vi "Date_request.vi"(8 "error in (no error)":errorcluster, 10 "SQL request":string, 11 "DB_SQLite in":refnum<class "DB_SQLite.lvclass">) -> (0 "error out":errorcluster, 2 "Date":timestamp, 3 "DB_SQLite out":refnum<class "DB_SQLite.lvclass">)   [LabVIEW 2015, in "DB_SQLite.lvclass"]
uses:
  DB_SQLite.lvclass
  <vilib>/drjdpowell/SQLite Library/SQL Connection/Connection.lvclass
  <vilib>/drjdpowell/SQLite Library/SQL Connection/Open (path).vi
  <vilib>/drjdpowell/SQLite Library/SQLite.lvlib
  DB.lvclass
  <vilib>/drjdpowell/SQLite Library/SQL Connection/Execute SQL (No results).vi
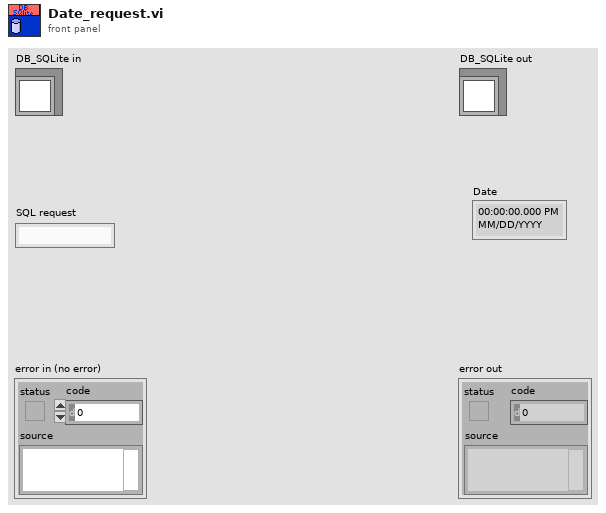
[diagram p1: front panel]
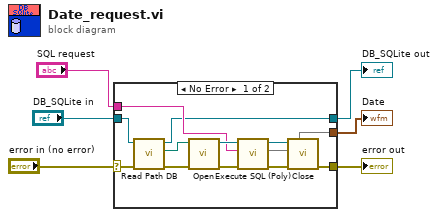
[diagram p0: block diagram]
diagram:
  n1 = case shown="No Error" "error in (no error)" {
    selector: "error in (no error)" -> [w10 w19]
    tunnel: [w7 w20] -> w5
    tunnel: "DB_SQLite in" -> [w11 w20]
    tunnel: "SQL request" -> [w14 _]
    tunnel: [w13 _] -> w2
    tunnel: [w12 w19] -> w1
    frame No Error {
      n2 = call "Read Path DB.vi"("error in (no error)"=w10, "DB in"=w11) -> ("error out"=w9:errorcluster, "Path DB"=w8:path, "DB out"=w7:refnum<class "DB_SQLite.lvclass">)  [unwired: 7 in]
      n3 = call-poly <vilib>:"Open.vi"("error in (no error)"=w9, "db file"=w8) -> ("error out"=w15:errorcluster, "SQLite Connection"=w16:refnum<class "Connection.lvclass">)  [unwired: 8 in]
      n4 = call-poly <vilib>:"Execute SQL (Poly).vi"("error in (no error)"=w15, "SQL"=w14, "SQLite Connection in"=w16) -> ("error out"=w18:errorcluster, 2:w13, "SQLite Connection"=w17:refnum<class "Connection.lvclass">)  [unwired: 6 in]
      n5 = call-dynamic "Close.vi"("error in (no error)"=w18, "SQLite Connection in"=w17) -> ("error out"=w12:errorcluster)  [unwired: 9 in]
    }
    frame Error {
    }
  }
  "error out" <- w1
  "DB_SQLite out" <- w5
  "Date" <- w2
